vi "GetSVLibraryFromDeviceName.vi"(8 "error in (no error)":errorcluster, 11 "DeviceName":string) -> (0 "error out":errorcluster, 2 "Current Variables":string[](array[string]), 3 "Open Library Reference":refnum<vi>, 5 "Library Path":path, 7 "Application Reference":refnum<vi>)   [LabVIEW 2013]
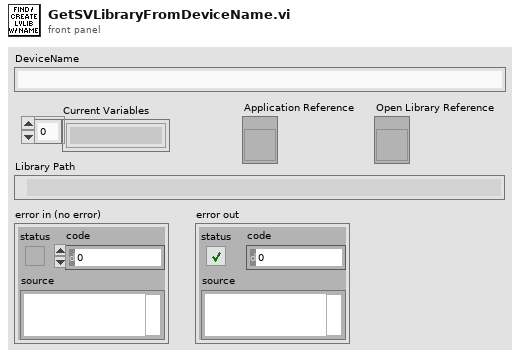
[diagram p1: front panel]
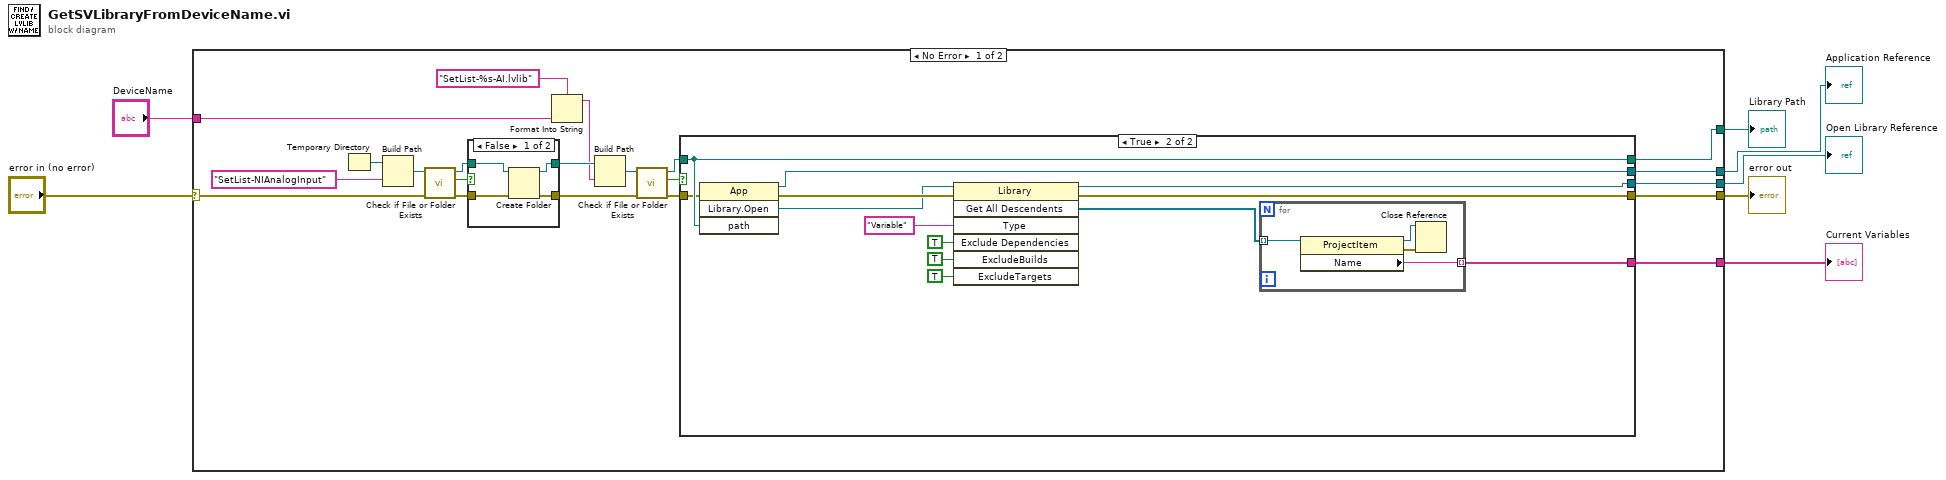
[diagram p0: block diagram]
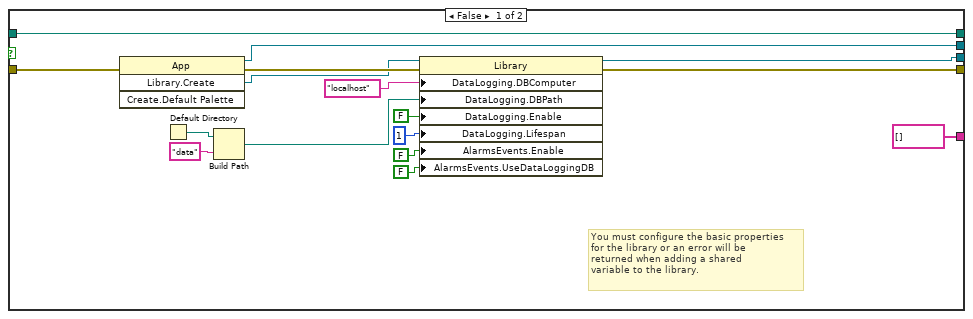
[diagram p2: hidden frame]
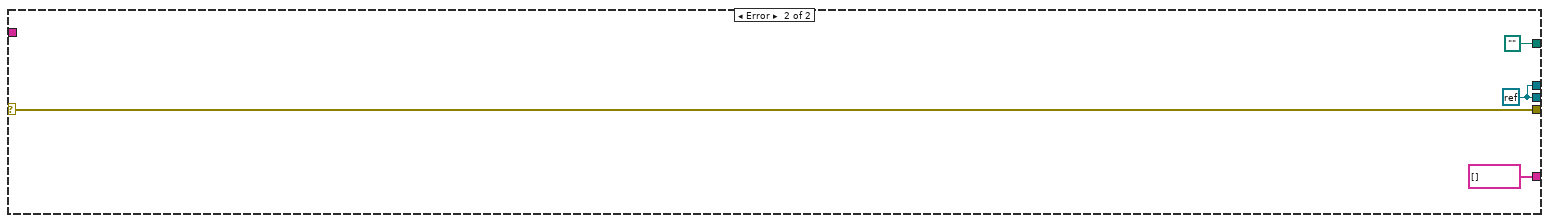
[diagram p4: hidden frame]
diagram:
  n1 = case shown="No Error" "error in (no error)" {
    selector: "error in (no error)" -> [w8 w71]
    tunnel: "DeviceName" -> [w28 _]
    tunnel: [w26 w71] -> w6
    tunnel: [w25 w68] -> w5
    tunnel: [w24 string[] []] -> w4
    tunnel: [w23 path ""] -> w3
    tunnel: [w14 w68] -> w2
    frame No Error {
      n2 = Temporary Directory() -> (w10:path)
      n3 = Build Path(base path=w10, name or relative path="SetList-NIAnalogInput") -> (appended path=w15:path)
      n4 = call <vilib>:"Check if File or Folder Exists.vi"("error in (no error)"=w8, "path"=w15) -> ("error out"=w20:errorcluster, "file or folder exists?"=w12:bool, "dup path"=w13:path)  [unwired: 7 in]
      n5 = case shown="False" w12 {
        tunnel: w13 -> [w65 w67]
        tunnel: [w64 w67] -> w19
        tunnel: w20 -> [w63 w66]
        tunnel: [w62 w66] -> w21
        frame False {
          n6 = Create Folder(path (use dialog)=w65, error in=w63) -> (created path=w64:path, error out=w62:errorcluster)  [unwired: 1 in, 1 out]
        }
        frame True {
        }
      }
      n7 = Format Into String(format string="SetList-%s-AI.lvlib", w28) -> (resulting string=w9:string)  [unwired: 2 in, 1 out]
      n8 = Build Path(base path=w19, name or relative path=w9) -> (appended path=w16:path)
      n9 = call <vilib>:"Check if File or Folder Exists.vi"("error in (no error)"=w21, "path"=w16) -> ("error out"=w22:errorcluster, "file or folder exists?"=w17:bool, "dup path"=w18:path)  [unwired: 7 in]
      n10 = case shown="True" w17 {
        tunnel: [w32 w45] -> w25
        tunnel: [w43 w57] -> w14
        tunnel: [w44 w56] -> w23
        tunnel: w18 -> [w44 w56]
        tunnel: w22 -> [w31 w55]
        tunnel: [w30 w47] -> w26
        tunnel: [string[] [] w49] -> w24
        frame False {
          # "You must configure the basic properties\nfor the library or an error will be\nreturned when adding a shared\nvariable to the library."
          n11 = invoke class="App" method="Library.Create"(error in=w31) -> (reference out=w43:refnum<vi>, error out=w34:errorcluster, "Create Library"=w33:refnum<vi>)  [unwired: 3 in, 1 out]
          n12 = Default Directory() -> (w40:path)
          n13 = Build Path(base path=w40, name or relative path="data") -> (appended path=w42:path)
          n14 = property class="Library"(reference=w33, error in=w34, "DataLogging.DBComputer"="localhost" ("AlarmsEvents:Database Computer"), "DataLogging.DBPath"=w42, "DataLogging.Enable"=FALSE ("DataLogging:Enable"), "DataLogging.Lifespan"=u32 1 ("DataLogging:Lifespan"), "AlarmsEvents.Enable"=FALSE ("AlarmsEvents:Enable"), "AlarmsEvents.UseDataLoggingDB"=FALSE ("AlarmsEvents:Use DataLogging Database")) -> (reference out=w32:refnum<vi>, error out=w30:errorcluster)
        }
        frame True {
          n15 = invoke class="App" method="Library.Open"(error in=w55, "path"=w56) -> (reference out=w57:refnum<vi>, error out=w48:errorcluster, "Open Library"=w46:refnum<vi>)  [unwired: 2 in, 1 out]
          n16 = invoke class="Library" method="Get All Descendents"(reference=w46, error in=w48, "Type"="Variable", "Exclude Dependencies"=TRUE ("ExcludeDependencies"), "ExcludeBuilds"=TRUE, "ExcludeTargets"=TRUE) -> (reference out=w45:refnum<vi>, error out=w47:errorcluster, "All Descendents"=w54:refnum<vi>[])  [unwired: 1 in, 4 out]
          n17 = for {
            tunnel: w54 -> [w60] mode=indexing
            tunnel: [w61] -> w49 mode=indexing
            n18 = property class="ProjectItem"(reference=w60) -> (reference out=w59:refnum<vi>, error out=w58:errorcluster, "Name"=w61:string)  [unwired: 1 in]
            n19 = Close Reference(reference=w59, error in (no error)=w58) -> ()  [unwired: 1 out]
          }
        }
      }
    }
    frame Error {
      w68 = refnum<k0> refnum
    }
  }
  "error out" <- w6
  "Open Library Reference" <- w5
  "Current Variables" <- w4
  "Library Path" <- w3
  "Application Reference" <- w2
